vi "Image_Snap_Dual.vi"(8 "error in":errorcluster, 10 "input cluster":T1={"L16 Linear Actuator"="ASRL6::INSTR", "XE 1000 Pump"="COM10", "Camera1"="cam2", "Camera2"="cam3", "Img_Capt"=TRUE, "Actuator"=TRUE, "Pump"=TRUE, "Cam 1"=TRUE, "Cam 2"=TRUE, "Empty_Refill"=FALSE, "Crop"=TRUE, "Light intensity"=50, "Exposure Time"=1000.0, "Sample Name"="Test Sample", "Operator"="MRJ", "Calibration 1"=path "C:/Users/au540322/Desktop/IHS_Project/calibration/Test Calibration/Test Calibration_7/1Test Calibration_7_2019_06_07-23-38-32-452.PNG", "Calibration 2"=path "C:/Users/au540322/Desktop/IHS_Project/calibration/Test Calibration/Test Calibration_7/2Test Calibration_7_2019_06_07-23-38-32-415.PNG", "Framerate"=1, "Timeout Sample"=50, "Collection date"="First test samples", "Sample size threshold"=1, "Empty start"=1, "Command"="MRJ", "Station"="", "Species Name"="", "Other Notes"="", "Aperture"=enum."Item 0", "Image Process Queue Size"=500, "Image Save Queue Size"=500, "Overload threshold"=500, "Max Framerate"=100, "Rectangle 1"={"Left"=0, "Top"=0, "Right"=0, "Bottom"=0, "Rotation"=0.0}, "Rectangle 2"={"Left"=0, "Top"=0, "Right"=0, "Bottom"=0, "Rotation"=0.0}, "Detection Region %"=0.0, "Detect 1"=path "C:/Users/au540322/Desktop/IHS_Project/images/Debris/Debris_0/Debris_0_2019_06_01-23-32-49-686.PNG", "Detect 2"=path "C:/Users/au540322/Desktop/IHS_Project/images/Debris/Debris_0/Debris_0_2019_06_01-23-32-49-686.PNG", "Max large object threshold"=0, "Open(T)/Close(F)"=FALSE, "Img_Capt Begin"=FALSE, "Dispense Speed"=100, "Flush Size"=100, "Location"="Station", "Latitude"="Station", "Longitude"="Station", "Determiner"="Station", "Sex"="Station", "Camera1_Img"="remote image 0000000015E6FBB4", "Camera2_Img"="remote image 0000000015E6F134", "Img1_Orig_Disp"=refnum, "Img2_Orig_Disp"=refnum, "Img1_Orig_RGB"=refnum, "Img2_Orig_RGB"=refnum, "Blue_Plane_Extract"=refnum, "Subtracted_Plane"=refnum, "Img1_Binary"=refnum, "Img2_Binary"=refnum, "Crop_Mask"=refnum, "Img1_Save"=refnum, "Img2_Save"=refnum, "Img1_Cali_Full"=refnum, "Img2_Cali_Full"=refnum, "Img1_Cali_Detect"=refnum, "Img2_Cali_Detect"=refnum, "Cam 1 queue"=refnum, "Cam 2 queue"=refnum, "Cam 1 - save queue"=refnum, "Cam 2 - save queue"=refnum, "Overlay_Ring"=0, "SystemVersion"=0, "System Serial"="", "Legacy Cam Attributes"=FALSE} {"SystemVersion" items=["Standard", "XL"]; "Overlay_Ring" items=["Session Data", "Extended Setup", "Buffer", "Camera", "Dispenser", "Stats", "Connections"]; "Flush Size" min=1; "Dispense Speed" min=1; "Rectangle 2"."Rotation" format="%.2f"; "Rectangle 2"."Left" scale=0.0..1024.0; "Rectangle 2"."Right" scale=0.0..1024.0; "Rectangle 1"."Rotation" format="%.2f"; "Rectangle 1"."Left" scale=0.0..1024.0; "Rectangle 1"."Right" scale=0.0..1024.0; "Max Framerate" min=1; "Overload threshold" min=1; "Image Save Queue Size" min=1; "Image Process Queue Size" min=1; "Empty start" min=1; "Sample size threshold" min=1; "Framerate" min=1; "Light intensity" scale=0.0..100.0}, 11 "Detect Movement":bool) -> (1 "Image2":T4, 2 "Image1":T4, 3 "Framerate":i32)   [LabVIEW 2022 SP3]
doc: "Gather pictures from both cameras, returns two picture arrays."
uses:
  <vilib>/vision/Image Controls.llb/IMAQ Image.ctl
  controls/Data.ctl
  <vilib>/userdefined/High Color/IMAQdx.ctl
  <vilib>/vision/driver/IMAQdx.llb/IMAQdx Acquisition Mode.ctl
  Camera_ID.ctl
  <vilib>/vision/driver/NI_Vision_Acquisition_Software.lvlib
panel:
  in  "error in 2":errorcluster
  out "error out 2":errorcluster
  out "error out":errorcluster
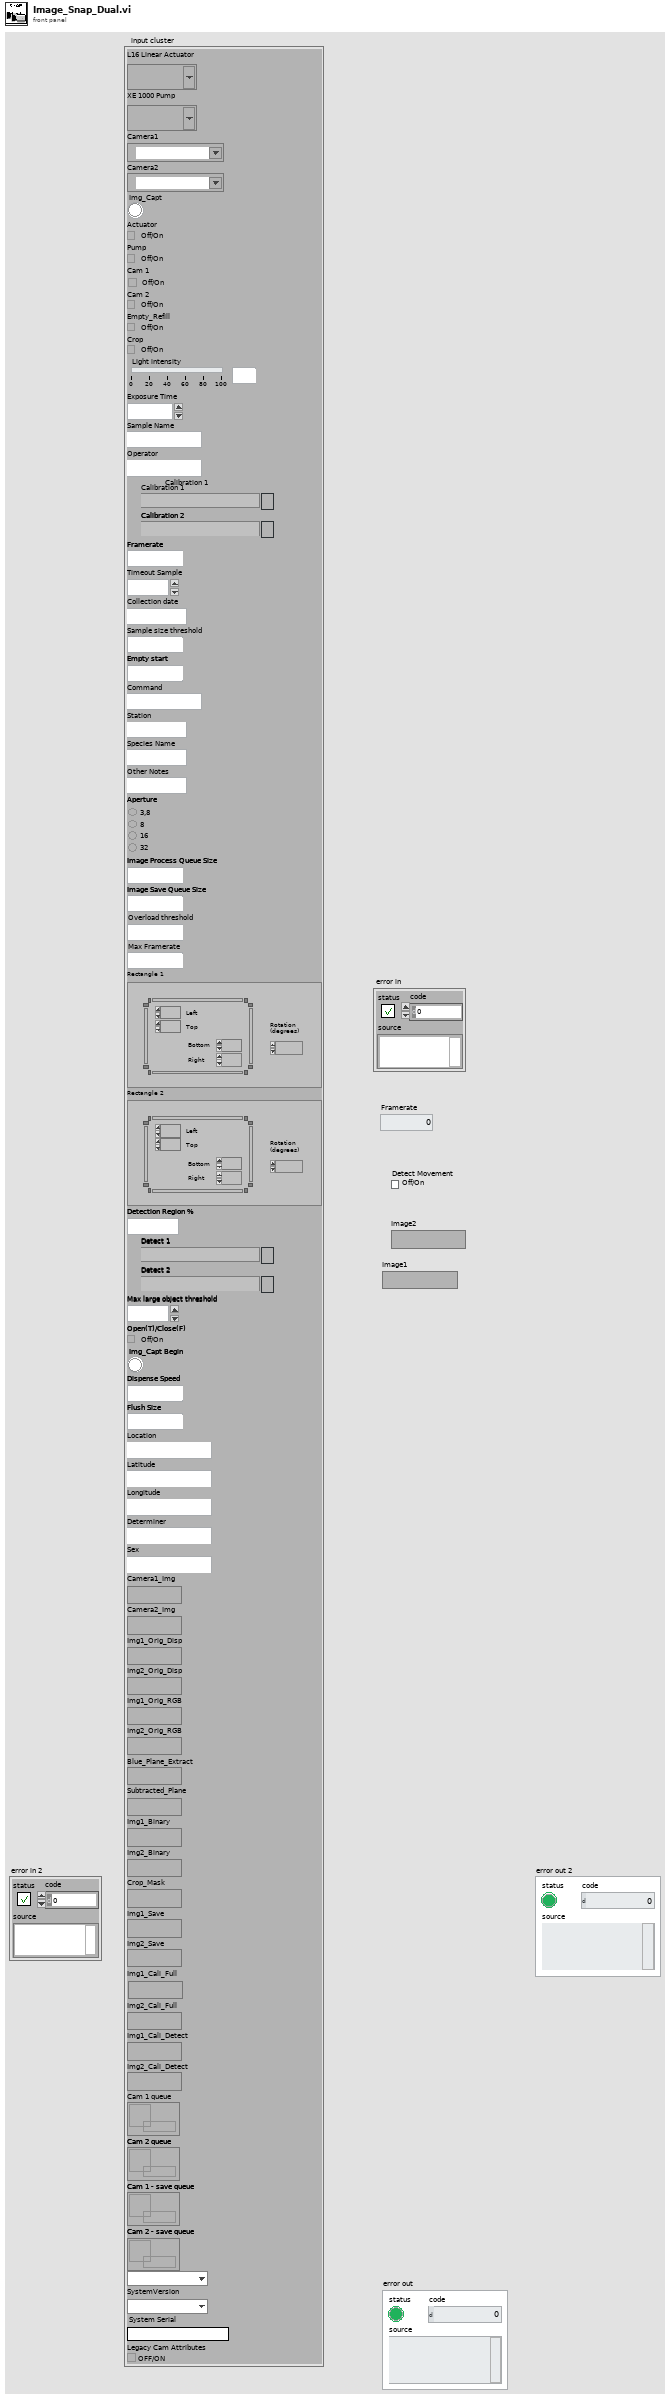
[diagram p1: front panel]
types:
  T1 = typedef "Data.ctl" = cluster{"L16 Linear Actuator":refnum<visa-resource-name>, "XE 1000 Pump":refnum<visa-resource-name>, "Camera1":T2, "Camera2":T2, "Img_Capt":bool, "Actuator":bool, "Pump":bool, "Cam 1":bool, "Cam 2":bool, "Empty_Refill":bool, "Crop":bool, "Light intensity":i32, "Exposure Time":dbl, "Sample Name":string, "Operator":string, "Calibration 1":path, "Calibration 2":path, "Framerate":i32, "Timeout Sample":i32, "Collection date":string, "Sample size threshold":i32, "Empty start":u32, "Command":string, "Station":string, "Species Name":string, "Other Notes":string, "Aperture":enum32{"Item 0", "Item 1", "Item 2", "Item 3"}, "Image Process Queue Size":i32, "Image Save Queue Size":i32, "Overload threshold":i32, "Max Framerate":i32, "Rectangle 1":T3, "Rectangle 2":T3, "Detection Region %":dbl, "Detect 1":path, "Detect 2":path, "Max large object threshold":i32, "Open(T)/Close(F)":bool, "Img_Capt Begin":bool, "Dispense Speed":i32, "Flush Size":i32, "Location":string, "Latitude":string, "Longitude":string, "Determiner":string, "Sex":string, "Camera1_Img":T4, "Camera2_Img":T4, "Img1_Orig_Disp":T4, "Img2_Orig_Disp":T4, "Img1_Orig_RGB":T4, "Img2_Orig_RGB":T4, "Blue_Plane_Extract":T4, "Subtracted_Plane":T4, "Img1_Binary":T4, "Img2_Binary":T4, "Crop_Mask":T4, "Img1_Save":T4, "Img2_Save":T4, "Img1_Cali_Full":T4, "Img2_Cali_Full":T4, "Img1_Cali_Detect":T4, "Img2_Cali_Detect":T4, "Cam 1 queue":refnum<queue>, "Cam 2 queue":refnum<queue>, "Cam 1 - save queue":refnum<queue>, "Cam 2 - save queue":refnum<queue>, "Overlay_Ring":u16, "SystemVersion":u16, "System Serial":string, "Legacy Cam Attributes":bool}
  T2 = typedef "IMAQdx.ctl" = refnum<k21>
  T3 = typedef "IMAQ Rectangle" = cluster{"Left":i32, "Top":i32, "Right":i32, "Bottom":i32, "Rotation":dbl}
  T4 = typedef "IMAQ Image.ctl" = refnum<image>
  T5 = typedef "NI_Vision_Acquisition_Software.lvlib/IMAQdx Acquisition Mode.ctl" = enum32{"One Shot", "Continuous"}
  T6 = typedef "Camera_ID.ctl" = enum16{"Camera 1", "Camera 2"}
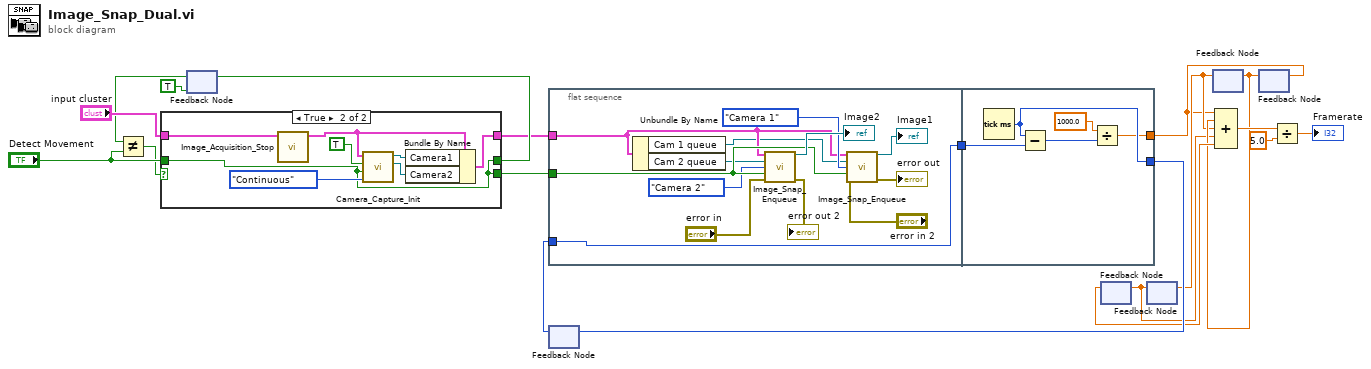
[diagram p0: block diagram]
diagram:
  n1 = feedback #1(TRUE ("Detect Movement")) -> (w6:bool)
  n2 = Not Equal?(x=w6, y="Detect Movement") -> (x != y?=w7:bool)
  n3 = case shown="True" w7 {
    tunnel: "input cluster" -> [w21 w23]
    tunnel: "Detect Movement" -> [w20 w24]
    tunnel: [w20 w24] -> w5
    tunnel: [w21 w25] -> w2
    tunnel: [w20 w24] -> w4
    frame False {
    }
    frame True {
      n4 = call "Image_Acquisition_Stop.vi"("input cluster"=w23) -> ("input cluster 2"=w22:T1)  [unwired: 9 in, 1 out]
      n5 = call "Camera_Capture_Init.vi"("Continuous?"=IMAQdx_Acquisition_Mode."Continuous", "Detect Movement"=w24, "Crop?"=TRUE, "input cluster"=w22) -> ("Camera2"=w26:T2, "Camera1"=w27:T2)  [unwired: 6 in]
      n6 = Bundle By Name(cluster=w22, "Camera1"=w27, "Camera2"=w26) -> (w25:T1)
    }
  }
  n7 = feedback-in #1(w5) -> ()
  n8 = flat-sequence {
    tunnel: [w39] -> w1
    tunnel: w18 -> [w39]
    tunnel: w2 -> [w35]
    tunnel: w4 -> [w38]
    tunnel: w1 -> [w47]
    tunnel: [w46] -> w19
    tunnel: [w43] -> w10
    frame #0 {
      n9 = Unbundle By Name(w35) -> ("Cam 1 queue"=w34:refnum<queue>, "Cam 2 queue"=w33:refnum<queue>)
      n10 = call "Image_Snap_Enqueue.vi"("input cluster"=w35, "Camera queue"=w33, "Camera"=Camera_ID."Camera 2", "Detect Movement"=w38, "error in"="error in") -> ("Image out"=→"Image2":T4, "error out"=→"error out 2":errorcluster)  [unwired: 9 in]
      n11 = call "Image_Snap_Enqueue.vi"("input cluster"=w35, "Camera queue"=w34, "Camera"=Camera_ID."Camera 1", "Detect Movement"=w38, "error in"="error in 2") -> ("Image out"=→"Image1":T4, "error out"=→"error out":errorcluster)  [unwired: 9 in]
    }
    frame #1 {
      n12 = Tick Count (ms)() -> (millisecond timer value=w46:u32)
      n13 = Subtract(x=w46, y=w47) -> (x-y=w45:u32)
      n14 = Divide(x=1000.0, y=w45) -> (x/y=w43:dbl)
    }
  }
  n15 = feedback #2() -> (w18:u32)  [unwired: 1 in]
  n16 = feedback-in #2(w19) -> ()
  n17 = feedback #3() -> (w14:dbl)  [unwired: 1 in]
  n18 = feedback #4() -> (w11:dbl)  [unwired: 1 in]
  n19 = feedback-in #3(w11) -> ()
  n20 = feedback #5() -> (w12:dbl)  [unwired: 1 in]
  n21 = feedback-in #4(w12) -> ()
  n22 = feedback #6() -> (w13:dbl)  [unwired: 1 in]
  n23 = feedback-in #5(w13) -> ()
  n24 = Compound Arithmetic op=ADD(w10, w13, w12, w11, w14) -> (w17:dbl)
  n25 = feedback-in #6(w10) -> ()
  n26 = Divide(x=w17, y=5.0) -> (x/y=→"Framerate":dbl)
